vi "test check cluster field names.vi"() -> ()   [LabVIEW 2018]
uses:
  LV-Julia_ZMQ-Roundtrip_lib.lvlib
panel:
  in  "Clout":T1(array[cluster])
  out "error out":errorcluster
  in  "error in (no error)":errorcluster
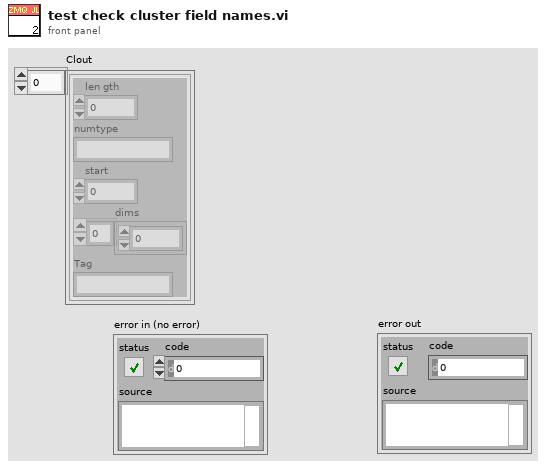
[diagram p1: front panel]
types:
  T1 = cluster{"len gth":i32, "numtype":string, "start":i32, "dims":i32[], "Tag":string}[]
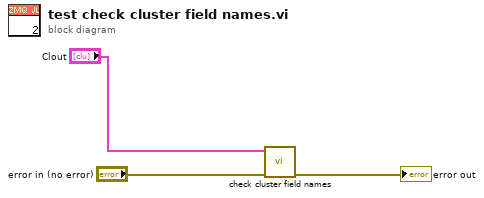
[diagram p0: block diagram]
diagram:
  n1 = call "check cluster field names.vi"("error in (no error)"="error in (no error)", "cluster or arr in"="Clout") -> ("error out"=→"error out":errorcluster)  [unwired: 9 in]
